vi "CLD 12 Sequencer State Machine.vi"() -> ()   [LabVIEW 2025]
doc: "CLD 12 exercise"
uses:
  CLD 12 Data Cluster.ctl
  CLD 12 Sequencer Enum.ctl
  CLD12 Timer Enum.ctl
  <vilib>/ErrorRing/Error Ring.xnode
panel:
  out "Current Time Target":dbl
  in  "Stop Button":bool
  out "Time Elapsed":dbl
  out "Switch 3":bool
  out "Switch 2":bool
  out "Switch 1":bool
  in  "Start":bool
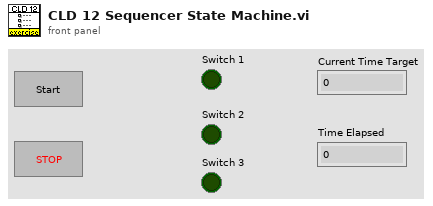
[diagram p1: front panel]
types:
  T1 = typedef "CLD 12 Data Cluster.ctl" = cluster{"Command":T2, "Time Value":dbl, "Boolean":bool, "Boolean 2":bool, "Boolean 3":bool}
  T2 = typedef "CLD 12 Sequencer Enum.ctl" = enum16{"Initialize", "SetTime", "RunState1", "Runstate2", "Idle", "Start"}
  T3 = typedef "CLD12 Timer Enum.ctl" = enum16{"Start Timer", "Read Time", "Pause", "UnPause", "Reset Timer"}
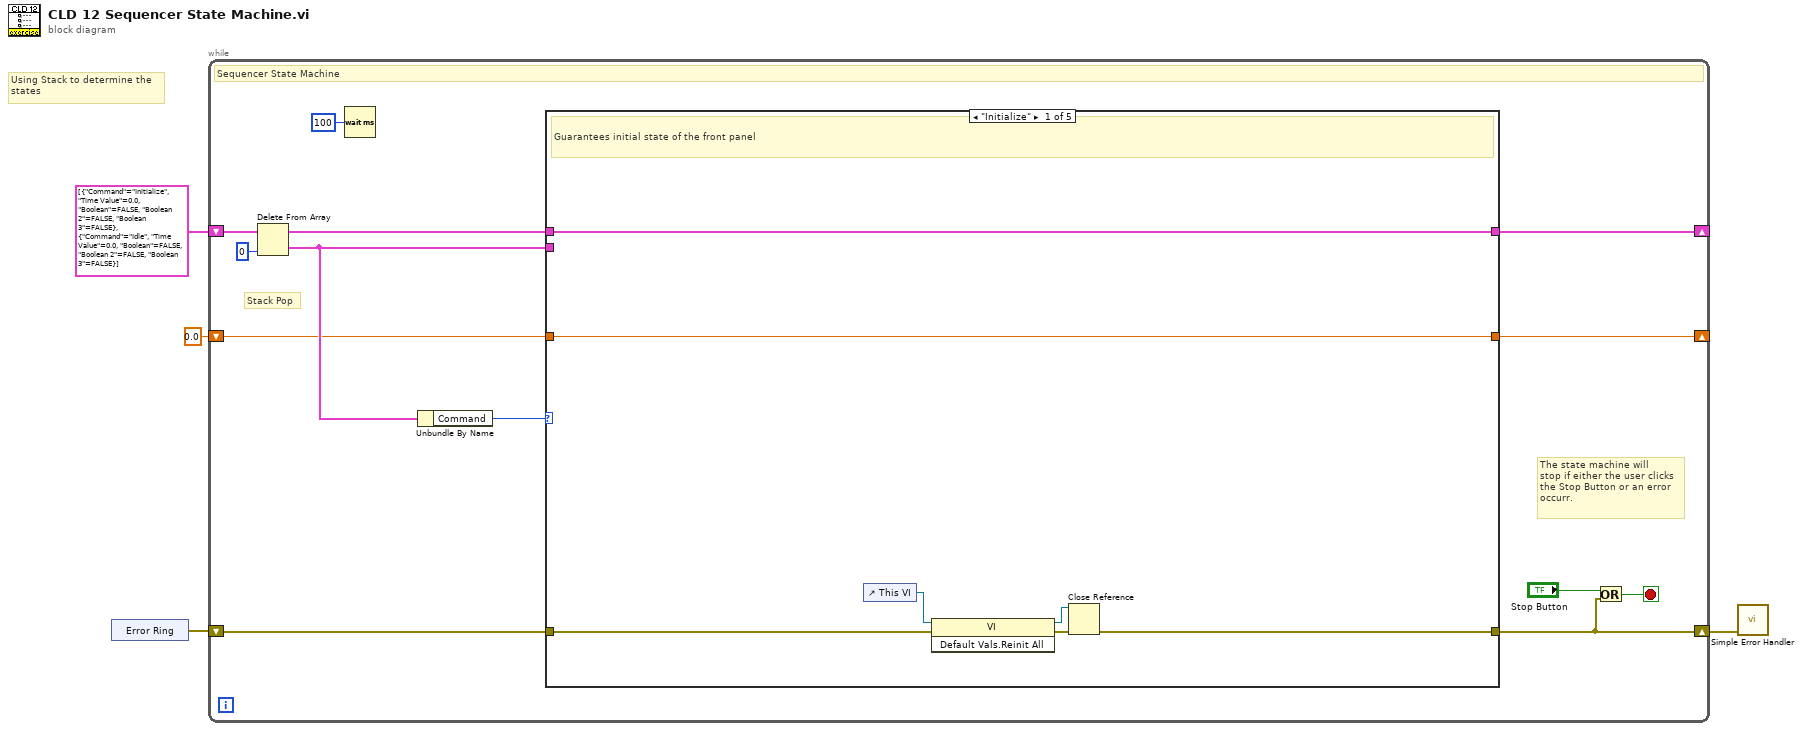
[diagram p0: block diagram]
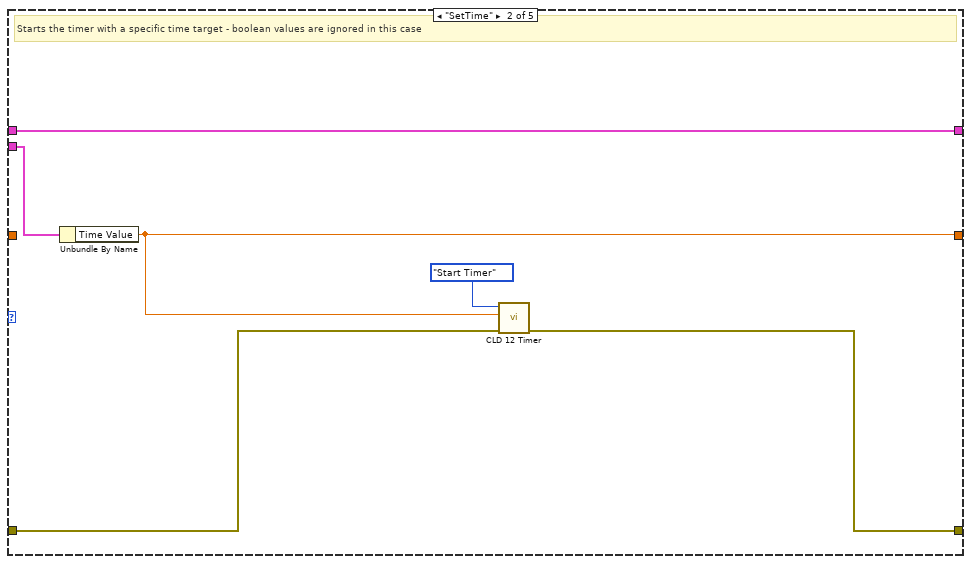
[diagram p2: hidden frame]
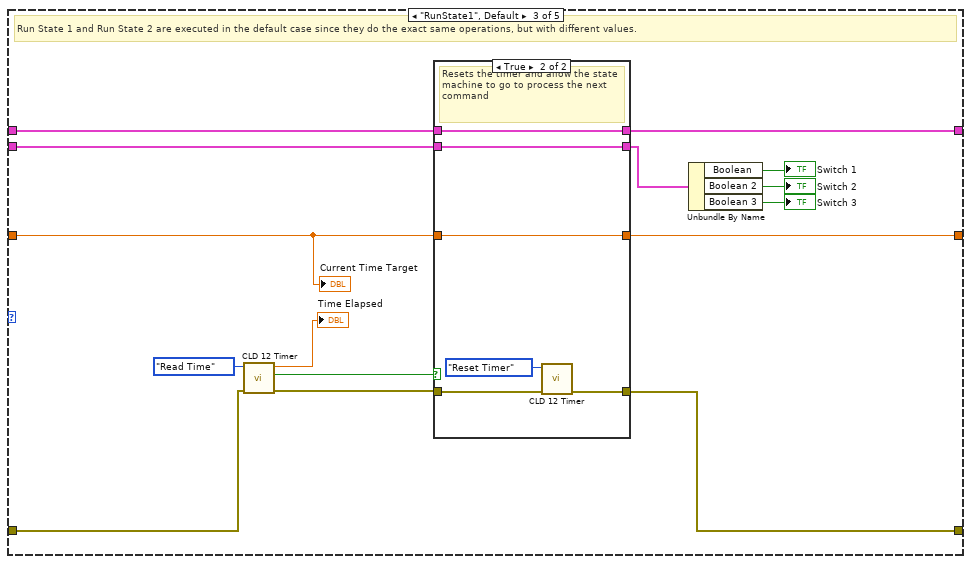
[diagram p3: hidden frame]
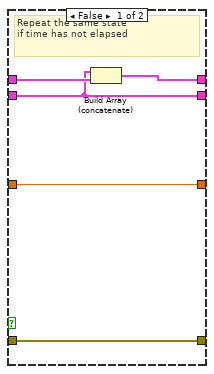
[diagram p4: hidden frame]
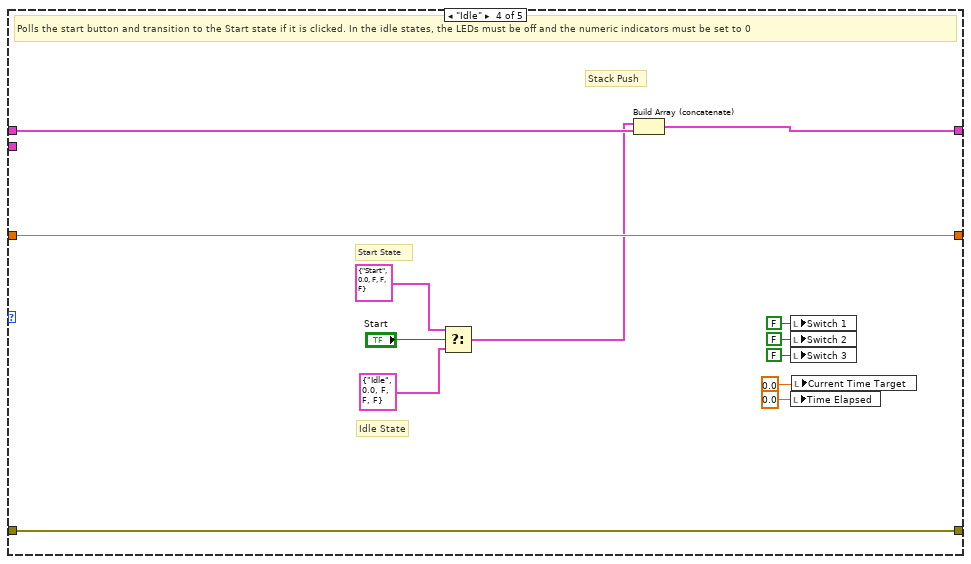
[diagram p5: hidden frame]
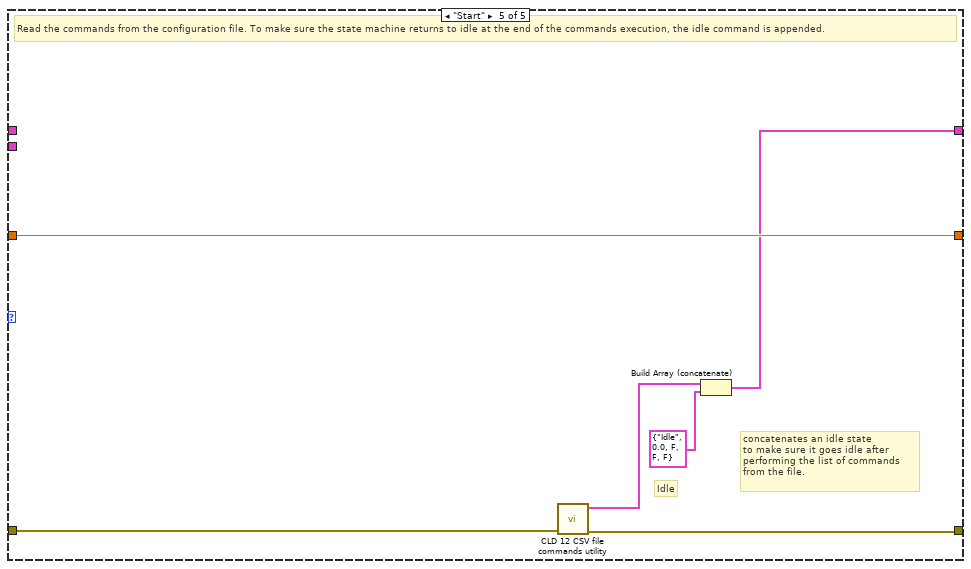
[diagram p6: hidden frame]
diagram:
  # "Using Stack to determine the\nstates"
  n1 = xnode "Error Ring"() -> ("error out"=w4:errorcluster)
  n2 = while {
    shift-right: [w9] -> w1
    shift-left: w4 -> [w16]
    shift-right: [w15] -> _
    shift-left: T1[] [{"Command"=enum."Initialize", "Time Value"=0.0, "Boolean"=FALSE, "Boolean 2"=FALSE, "Boolean 3"=FALSE}, {"Command"=enum."Idle", "Time Value"=0.0, "Boolean"=FALSE, "Boolean 2"=FALSE, "Boolean 3"=FALSE}] ("Array") -> [w17]
    shift-right: [w6] -> _
    shift-left: 0.0 ("Time Value") -> [w8]
    stop <- w10 stop-if-true
    # "The state machine will\nstop if either the user clicks\nthe Stop Button or an error\noccurr."
    # "Stack Pop"
    # "Sequencer State Machine"
    n3 = Delete From Array "Delete From Array"(array=w17, index=0) -> (deleted portion=w12:T1, array with subset deleted=w14:T1[])  [unwired: 1 in]
    n4 = Wait (ms)(milliseconds to wait=u32 100) -> ()  [unwired: 1 out]
    n5 = Unbundle By Name(w12) -> ("Command"=w13:T2)
    n6 = case shown="\"Initialize\"" w13 {
      tunnel: w14 -> [w18 w30 w45 w68 _]
      tunnel: w16 -> [w20 w29 w44 w69 w74]
      tunnel: [w23 w27 w32 w69 w73] -> w9
      tunnel: [w18 w30 w41 w66 w70] -> w15
      tunnel: w12 -> [_ w26 w42 _ _]
      tunnel: [w19 w25 w35 w67 w75] -> w6
      tunnel: w8 -> [w19 _ w31 w67 w75]
      frame "Initialize" {
        # "Guarantees initial state of the front panel"
        n7 = control-ref of="This VI"() -> (w22:refnum<vi>)
        n8 = invoke class="VI" method="Default Vals.Reinit All"(reference=w22, error in=w20) -> (reference out=w24:refnum<vi>, error out=w21:errorcluster)  [unwired: 1 in, 1 out]
        n9 = Close Reference(reference=w24, error in (no error)=w21) -> (error out=w23:errorcluster)
      }
      frame "SetTime" {
        # "Starts the timer with a specific time target - boolean values are ignored in this case"
        n10 = Unbundle By Name(w26) -> ("Time Value"=w25:dbl)
        n11 = call "CLD 12 Timer.vi"("Error In"=w29, "Time Target (s)"=w25, "CLD 12 Timer Enum"=CLD12_Timer_Enum."Start Timer") -> ("Error Out"=w27:errorcluster)  [unwired: 6 in, 2 out]
      }
      frame "RunState1", Default {
        # "Run State 1 and Run State 2 are executed in the default case since they do the exact same operations, but with different values."
        n12 = call "CLD 12 Timer.vi"("Error In"=w44, "CLD 12 Timer Enum"=CLD12_Timer_Enum."Read Time") -> ("Error Out"=w33:errorcluster, "Has Time Elapsed ?"=w40:bool, "Elapsed Time (s.ss)"=→"Time Elapsed":dbl)  [unwired: 7 in]
        n13 = case shown="True" w40 {
          tunnel: w45 -> [w50 w56]
          tunnel: w42 -> [w47 w55]
          tunnel: w31 -> [w49 w54]
          tunnel: [w47 w55] -> w34
          tunnel: [w48 w56] -> w41
          tunnel: [w49 w54] -> w35
          tunnel: w33 -> [w46 w52]
          tunnel: [w46 w51] -> w32
          frame False {
            # "Repeat the same state\nif time has not elapsed"
            n14 = Build Array (concatenate)(w47, w50) -> (w48:T1[])
          }
          frame True {
            # "Resets the timer and allow the state machine to go to process the next command"
            n15 = call "CLD 12 Timer.vi"("Error In"=w52, "CLD 12 Timer Enum"=CLD12_Timer_Enum."Reset Timer") -> ("Error Out"=w51:errorcluster)  [unwired: 7 in, 2 out]
          }
        }
        n16 = Unbundle By Name(w34) -> ("Boolean"=→"Switch 1":bool, "Boolean 2"=→"Switch 2":bool, "Boolean 3"=→"Switch 3":bool)
        "Current Time Target" <- w31
      }
      frame "Idle" {
        # "Idle State"
        # "Start State"
        # "Stack Push"
        # "Polls the start button and transition to the Start state if it is clicked. In the idle states, the LEDs must be off and the numeric indicators must be set to 0"
        n17 = Select(t=T1 {"Command"=enum."Start", "Time Value"=0.0, "Boolean"=FALSE, "Boolean 2"=FALSE, "Boolean 3"=FALSE} ("CLD 12 Data Cluster"), s="Start", f=T1 {"Command"=enum."Idle", "Time Value"=0.0, "Boolean"=FALSE, "Boolean 2"=FALSE, "Boolean 3"=FALSE} ("CLD 12 Data Cluster")) -> (s? t:f=w62:T1)
        n18 = Build Array (concatenate)(w62, w68) -> (w66:T1[])
        n19 = local write "Switch 1"(FALSE ("Switch 1")) -> ()
        n20 = local write "Switch 2"(FALSE ("Switch 2")) -> ()
        n21 = local write "Switch 3"(FALSE ("Switch 3")) -> ()
        n22 = local write "Time Elapsed"(0.0 ("Time Elapsed")) -> ()
        n23 = local write "Current Time Target"(0.0 ("Current Time Target")) -> ()
      }
      frame "Start" {
        # "concatenates an idle state\nto make sure it goes idle after\nperforming the list of commands\nfrom the file."
        # "Idle"
        # "Read the commands from the configuration file. To make sure the state machine returns to idle at the end of the commands execution, the idle command is appended."
        n24 = call "CLD 12 CSV file commands utility.vi"("Error In"=w74) -> ("Error Out"=w73:errorcluster, "Command Array Out"=w72:T1[])  [unwired: 9 in]
        n25 = Build Array (concatenate)(w72, T1 {"Command"=enum."Idle", "Time Value"=0.0, "Boolean"=FALSE, "Boolean 2"=FALSE, "Boolean 3"=FALSE} ("CLD 12 Data Cluster")) -> (w70:T1[])
      }
    }
    n26 = Or(x="Stop Button", y=w9) -> (x .or. y?=w10:bool)
  }
  n27 = call <vilib>:"Simple Error Handler.vi"("error in (no error)"=w1) -> ()  [unwired: 4 in, 5 out]
